vi "Set_Get Target Info.vi"(8 "error in (no error)":errorcluster, 10 "Hardware Version":T1, 11 "IP Address (format: IP Address or DNS Name)":string) -> (0 "error out":errorcluster, 2 "Hardware Version":T1, 3 "IP Address":string)   [LabVIEW 2021]
uses:
  <vilib>/myRIO/Common/Instrument Driver Framework/Utilities/typedefs/Hardware Version Enum.ctl
panel:
  # "This VI is used to Set and Get the myRIO Target Information when attempting to run the myRIO API on a Desktop. The IP address is the IP address of the the myRIO target and the Hardware Version is the version of the myRIO target.\n\nIf you wish to run code on the Desktop and use the myRIO for sensor acquisition this VI MUST be run before any of the myRIO VIs otherwise they will fail.\n\nIf you are running the myRIO VIs in the Real-Time context (actually running the code on the target) then this VI is not necessary."
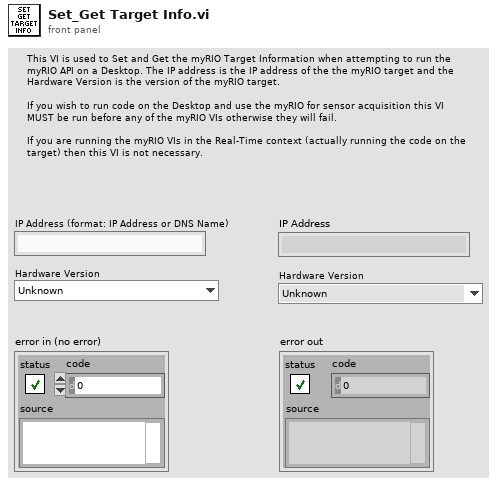
[diagram p1: front panel]
types:
  T1 = typedef "Hardware Version Enum.ctl" = enum16{"Unknown", "myRIO-1900", "myRIO-1950", "roboRIO", "NI ELVIS RIO CM", "ELVIS III"}
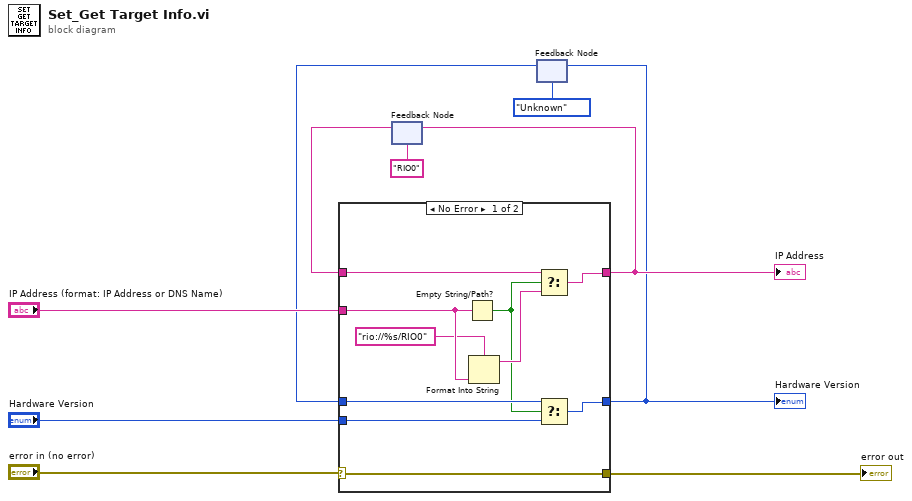
[diagram p0: block diagram]
diagram:
  n1 = feedback #1("RIO0") -> (w7:string)
  n2 = feedback #2(Hardware_Version_Enum."Unknown" ("Hardware Version")) -> (w6:T1)
  n3 = case shown="No Error" "error in (no error)" {
    selector: "error in (no error)" -> [w11 w21]
    tunnel: "IP Address (format: IP Address or DNS Name)" -> [w20 _]
    tunnel: w7 -> [w18 w23]
    tunnel: w6 -> [w17 w22]
    tunnel: [w16 w22] -> w3
    tunnel: [w15 w23] -> w4
    tunnel: "Hardware Version" -> [w13 _]
    tunnel: [w11 w21] -> w1
    frame No Error {
      n4 = Empty String/Path?(string/path=w20) -> (empty?=w12:bool)
      n5 = Format Into String(format string="rio://%s/RIO0", w20) -> (resulting string=w14:string)  [unwired: 2 in, 1 out]
      n6 = Select(t=w18, s=w12, f=w14) -> (s? t:f=w15:string)
      n7 = Select(t=w17, s=w12, f=w13) -> (s? t:f=w16:T1)
    }
    frame Error {
    }
  }
  "IP Address" <- w4
  "Hardware Version" <- w3
  "error out" <- w1
  n8 = feedback-in #1(w4) -> ()
  n9 = feedback-in #2(w3) -> ()
